vi "AutoAdjustGraphAspectRatio.vi"(11 "IntensityGraph in":refnum<vi>) -> ()   [LabVIEW 2017]
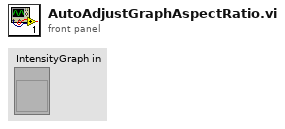
[diagram p1: front panel]
types:
  T1 = typedef "LVRectTypeDef.ctl" = cluster{"Left":i16, "Top":i16, "Right":i16, "Bottom":i16}
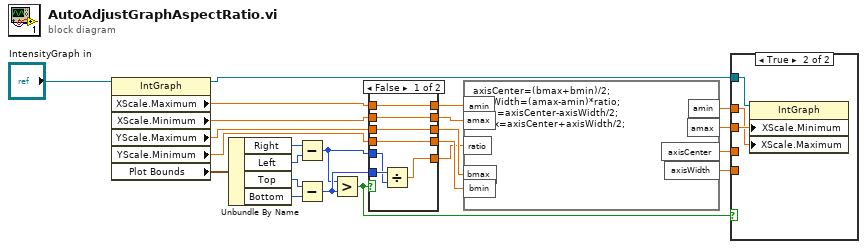
[diagram p0: block diagram]
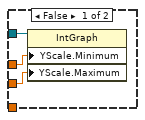
[diagram p2: hidden frame]
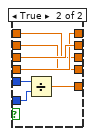
[diagram p3: hidden frame]
diagram:
  n1 = property on="Property Node" class="IntGraph"(reference="IntensityGraph in") -> (reference out=w11:refnum<vi>, "XScale.Maximum"=w8:dbl, "XScale.Minimum"=w9:dbl, "YScale.Maximum"=w3:dbl, "YScale.Minimum"=w5:dbl, "Plot Bounds"=w14:T1)  [unwired: 1 in, 1 out]
  n2 = Unbundle By Name(w14) -> ("Right"=w16:i16, "Left"=w15:i16, "Top"=w17:i16, "Bottom"=w18:i16)
  n3 = Subtract(x=w16, y=w15) -> (x-y=w19:i16)
  n4 = Subtract(x=w17, y=w18) -> (x-y=w20:i16)
  n5 = Greater?(x=w19, y=w20) -> (0:w10:bool)
  n6 = case shown="False" w10 {
    tunnel: w20 -> [w30 w37]
    tunnel: w19 -> [w29 w36]
    tunnel: w3 -> [w25 w35]
    tunnel: [w26 w35] -> w4
    tunnel: w5 -> [w24 w34]
    tunnel: [w27 w34] -> w6
    tunnel: [w28 w33] -> w7
    tunnel: w8 -> [w27 w32]
    tunnel: w9 -> [w26 w31]
    tunnel: [w25 w32] -> w21
    tunnel: [w24 w31] -> w22
    frame False {
      n7 = Divide(x=w30, y=w29) -> (x/y=w28:dbl)
    }
    frame True {
      n8 = Divide(x=w36, y=w37) -> (x/y=w33:dbl)
    }
  }
  n9 = formula code="axisCenter=(bmax+bmin)/2;\naxisWidth=(amax-amin)*ratio;\namin=axisCenter-axisWidth/2;\namax=axisCenter+axisWidth/2;"("amin"=w6, "amax"=w4, "ratio"=w7, "bmax"=w21, "bmin"=w22) -> ("amin"=w1:dbl, "amax"=w2:dbl, "axisCenter"=w13:dbl, "axisWidth"=w12:dbl)
  n10 = case shown="True" w10 {
    tunnel: w1 -> [w39 w41]
    tunnel: w2 -> [w38 w42]
    tunnel: w11 -> [w40 w43]
    tunnel: w12 -> [_ _]
    tunnel: w13 -> [_ _]
    frame False {
      n11 = property on="Property Node" class="IntGraph"(reference=w40, "YScale.Minimum"=w39, "YScale.Maximum"=w38) -> ()  [unwired: 1 in, 2 out]
    }
    frame True {
      n12 = property on="Property Node" class="IntGraph"(reference=w43, "XScale.Minimum"=w42, "XScale.Maximum"=w41) -> ()  [unwired: 1 in, 2 out]
    }
  }
